vi "move.vi"(8 "error in (no error)":errorcluster, 11 "DL090409StageScaffold in":refnum<class "StageDL090409Scaffold.lvclass">) -> (0 "error out":errorcluster, 3 "DL090409StageScaffold out":refnum<class "StageDL090409Scaffold.lvclass">)   [LabVIEW 2010, in "StageDL090409Scaffold.lvclass"]
uses:
  StageDL090409Scaffold.lvclass
  GenericStage/GenericStage/translation_mode_enum.ctl
  GenericStage/GenericStage/GenericStage.lvclass
  common/classes/SpaceVector/SpaceVector/SpaceVector.lvclass
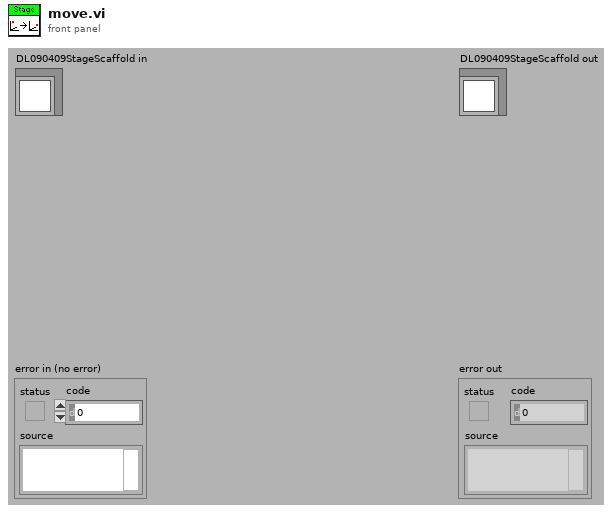
[diagram p1: front panel]
types:
  T1 = typedef "GenericStage.lvclass/translation_mode_enum.ctl" = enum16{"DON'T MOVE", "relative", "absolute"}
  T2 = typedef "GenericStage.lvclass/translation_request.ctl" = cluster{"translation mode":T1, "translation vector":refnum<class "SpaceVector.lvclass">}
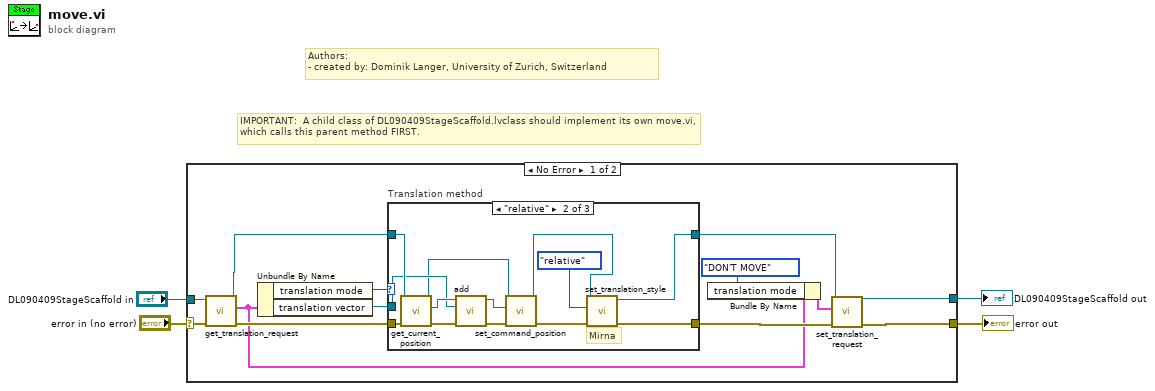
[diagram p0: block diagram]
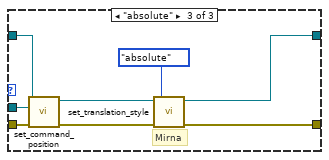
[diagram p3: hidden frame]
diagram:
  # "IMPORTANT:  A child class of DL090409StageScaffold.lvclass should implement its own move.vi, which calls this parent method FIRST."
  # "Authors: \n- created by: Dominik Langer, University of Zurich, Switzerland"
  n1 = case shown="No Error" "error in (no error)" {
    selector: "error in (no error)" -> [w17 w42]
    tunnel: [w16 w42] -> w3
    tunnel: [w6 w41] -> w1
    tunnel: "DL090409StageScaffold in" -> [w13 w41]
    frame No Error {
      n2 = call-dynamic "get_translation_request.vi"("error in (no error)"=w17, "GenericStage.lvclass in"=w13) -> ("error out"=w11:errorcluster, "translation request"=w7:T2, "GenericStage.lvclass out"=w12:refnum<class "StageDL090409Scaffold.lvclass">)  [unwired: 7 out]
      n3 = Unbundle By Name(w7) -> ("translation mode"=w5:T1, "translation vector"=w10:refnum<class "SpaceVector.lvclass">)
      n4 = case "Translation method" shown="\"relative\"" w5 {
        tunnel: w12 -> [w18 w31 w38]
        tunnel: w11 -> [w19 w32 w40]
        tunnel: w10 -> [_ w28 w39]
        tunnel: [w19 w22 w36] -> w9
        tunnel: [w18 w24 w33] -> w8
        frame "DON'T MOVE", Default {
        }
        frame "relative" {
          # "Mirna"
          n5 = call-dynamic "get_current_position.vi"("error in (no error)"=w32, "DL090409StageScaffold.lvclass in"=w31) -> ("error out"=w30:errorcluster, "current position"=w29:refnum<class "SpaceVector.lvclass">, "DL090409StageScaffold.lvclass out"=w25:refnum<class "StageDL090409Scaffold.lvclass">)  [unwired: 7 out]
          n6 = call "add.vi"("error in (no error)"=w30, "vector to be added"=w28, "SpaceVector in"=w29) -> ("error out"=w27:errorcluster, "SpaceVector out"=w26:refnum<class "SpaceVector.lvclass">)  [unwired: 7 out]
          n7 = call-dynamic "set_command_position.vi"("error in (no error)"=w27, "command position"=w26, "DL090409StageScaffold.lvclass in"=w25) -> ("error out"=w23:errorcluster, "DL090409StageScaffold.lvclass out"=w21:refnum<class "StageDL090409Scaffold.lvclass">)  [unwired: 7 out]
          n8 = call-dynamic "set_translation_style.vi"("error in (no error)"=w23, "translation style"=enum16{"relative", "absolute"}."relative", "StageDL090409Scaffold in"=w21) -> ("error out"=w22:errorcluster, "StageDL090409Scaffold out"=w24:refnum<class "StageDL090409Scaffold.lvclass">)  [unwired: 7 in]
        }
        frame "absolute" {
          # "Mirna"
          n9 = call-dynamic "set_command_position.vi"("error in (no error)"=w40, "command position"=w39, "DL090409StageScaffold.lvclass in"=w38) -> ("error out"=w37:errorcluster, "DL090409StageScaffold.lvclass out"=w34:refnum<class "StageDL090409Scaffold.lvclass">)  [unwired: 7 out]
          n10 = call-dynamic "set_translation_style.vi"("error in (no error)"=w37, "translation style"=enum16{"relative", "absolute"}."absolute", "StageDL090409Scaffold in"=w34) -> ("error out"=w36:errorcluster, "StageDL090409Scaffold out"=w33:refnum<class "StageDL090409Scaffold.lvclass">)  [unwired: 7 in]
        }
      }
      n11 = Bundle By Name(cluster=w7, "translation mode"=translation_mode_enum."DON'T MOVE") -> (w15:T2)
      n12 = call-dynamic "set_translation_request.vi"("error in (no error)"=w9, "translation request"=w15, "GenericStage.lvclass in"=w8) -> ("error out"=w16:errorcluster, "GenericStage.lvclass out"=w6:refnum<class "StageDL090409Scaffold.lvclass">)  [unwired: 7 out]
    }
    frame Error {
    }
  }
  "error out" <- w3
  "DL090409StageScaffold out" <- w1
